vi "Gold.vi"(7 "p":i32) -> (8 "I":cdb[](array[numeric]))   [LabVIEW 2017]
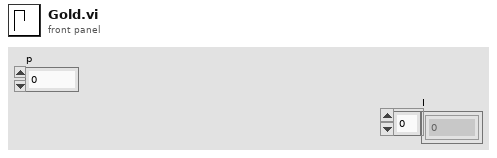
[diagram p1: front panel]
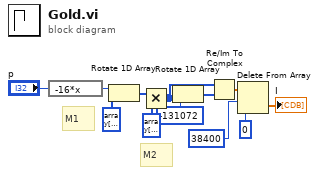
[diagram p0: block diagram]
diagram:
  # "M2"
  # "M1"
  n1 = expression code="-16*x"("p") -> (w1:i32)
  n2 = Rotate 1D Array(1:i32[] array[262143 elements] ("M1 2"), 2:w1) -> (0:w12:i32[])
  n3 = Multiply(x=w12, y=i32[] array[262143 elements] ("M2 2")) -> (x*y=w3:i32[])
  n4 = Rotate 1D Array(1:w3, 2:-131072 ("n")) -> (0:w10:i32[])
  n5 = Re/Im To Complex(1:w10, 2:w3) -> (0:w4:cdb[])
  n6 = Delete From Array(array=w4, length=38400, index=0) -> (deleted portion=→"I":cdb[])  [unwired: 1 out]
